vi "Create or Load Experiment Dialog.vi"(8 "error in (no error)":errorcluster) -> (0 "error out":errorcluster, 1 "Cancelled?":bool, 2 "Experimental File Cluster":T1, 3 "Experiment File Path":path, 4 "Experiment File Extension":string, 5 "Experiment Name":string)   [LabVIEW 2020, in "Experiment Manager.lvlib"]
uses:
  Experiment Manager.lvlib
  Experiment File/Experiment File Cluster.ctl
  Plugin Servers/Controller/Minimal Controller Cluster.ctl
  Plugin Servers/Parameter to Hardware Map/Minimal Map.ctl
  Plugin Servers/Parameter to Hardware Map/Minimal Pair Cluster.ctl
  UI Data.ctl
  User Preferences/User Preferences File.lvclass
  Sub VIs/Message Queue/Enqueue Message (Single).vi
  <vilib>/Utility/error.llb/Error Cluster From Error Code.vi
  <vilib>/ErrorRing/Error Ring.xnode
  Sub VIs/Message Queue/test Message Queue.lvlib
  User Event - Stop/User Event - Stop.lvlib
  Plugin Servers/Controller/Generic Plugin.lvclass
  Experiment File/Experiment File.lvlib
  Plugin Servers/Parameter to Hardware Map/Parameter to Hardware Map.lvclass
panel:
  in  "Continue Without Experiment Btn":bool
  in  "Load Experiment Btn":bool
  in  "New Experiment Btn":bool
  in  "Clear Recent Experiments Button":bool
  in  "Recent Experiments Listbox":i32(listbox)
  # "Create or Load Experiment"
  # "Experiment Options"
  # "Recent Experiments"
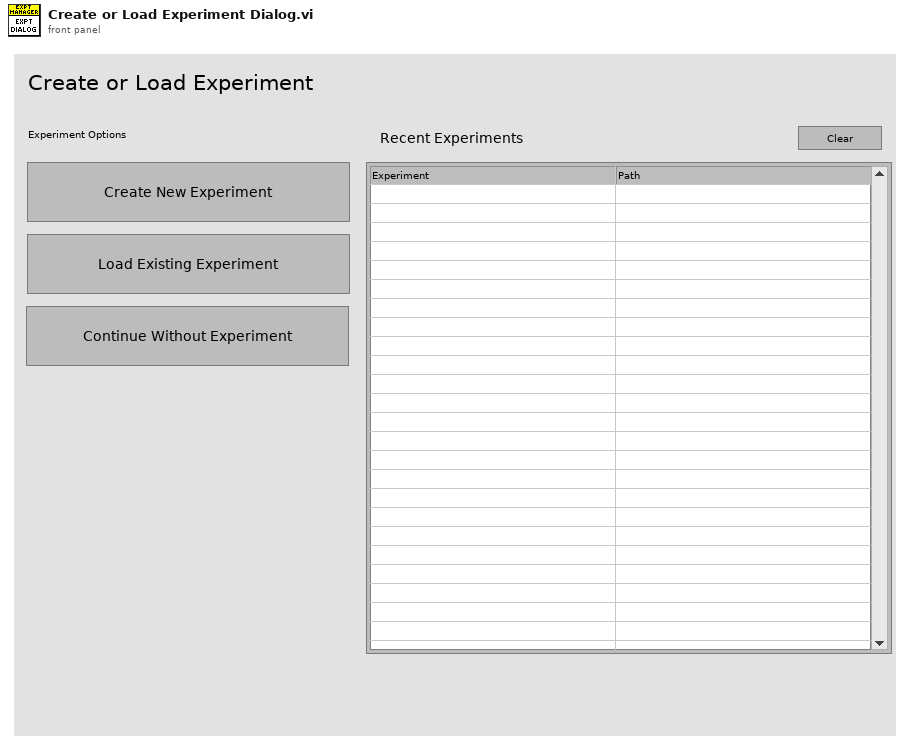
[diagram p1: front panel]
types:
  T1 = typedef "Experiment File.lvlib/Experiment File Cluster.ctl" = cluster{"Hardware List":T2[], "Optimizer List":T2[], "Analyzer List":T2[], "Parameter to Hardware Map":T3}
  T2 = typedef "Generic Plugin.lvclass/Minimal Controller Cluster.ctl" = cluster{"Name":string, "Controller Type":string, "Control Panel Path":string, "Resource":string}
  T3 = typedef "Parameter to Hardware Map.lvclass/Minimal Map.ctl" = T4[]
  T4 = typedef "Parameter to Hardware Map.lvclass/Minimal Pair Cluster.ctl" = cluster{"key":string, "values":T2[]}
  T5 = typedef "Experiment Manager.lvlib/UI Data.ctl" = cluster{"New Project Btn":refnum<vi>, "Load Project Btn":refnum<vi>, "Cancelled?":bool, "Experiment File Path":path, "Experiment File":T1, "Experiment Directory":path, "Experiment Name":string, "Experiment File Extension":string, "User Preferences File":refnum<class "User Preferences File.lvclass">, "Recent Experiments Listbox":refnum<vi>}
  T6 = enum32{"Invalid", "Standard", "Closed", "Hidden", "Minimized", "Maximized"}
  T7 = typedef "User Preferences File.lvclass/User Preferences Cluster.ctl" = cluster{"Max Recent Experiments":dbl, "Recent Experiments":string[]}
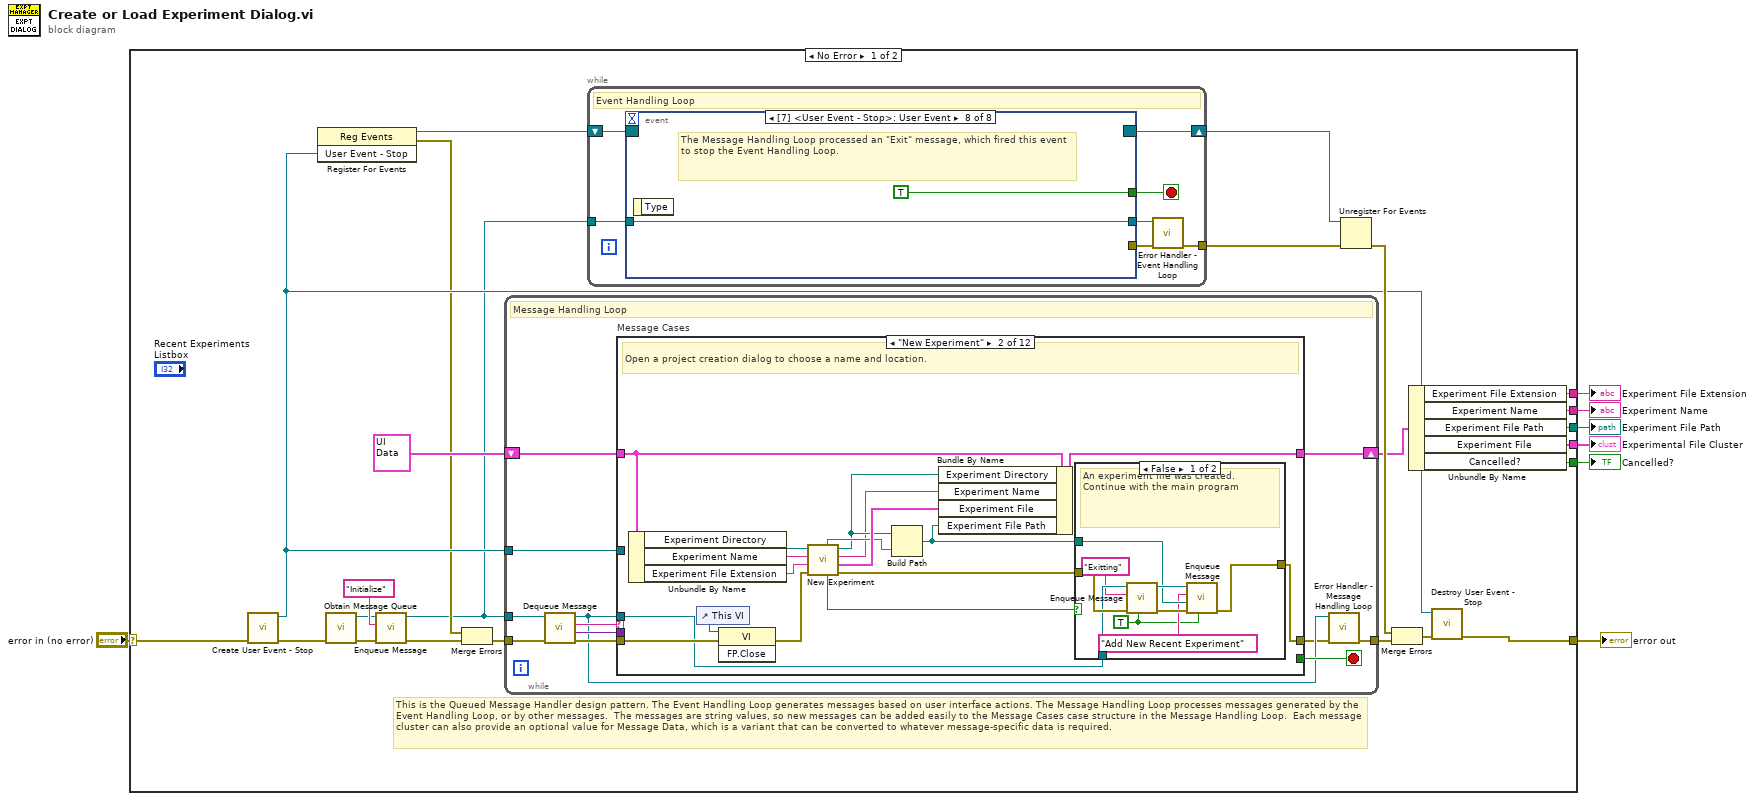
[diagram p0: block diagram]
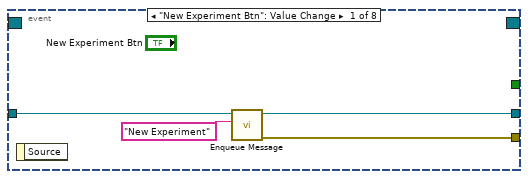
[diagram p2: hidden frame]
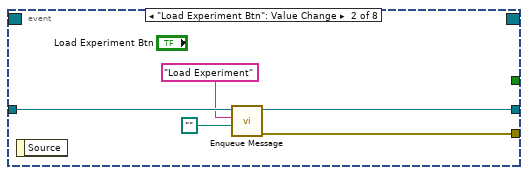
[diagram p3: hidden frame]
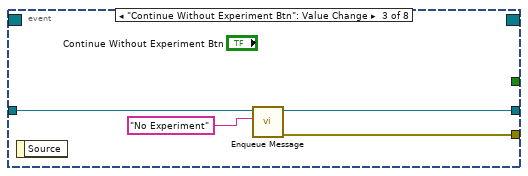
[diagram p4: hidden frame]
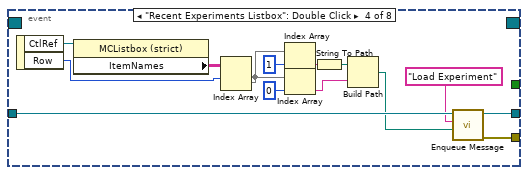
[diagram p5: hidden frame]
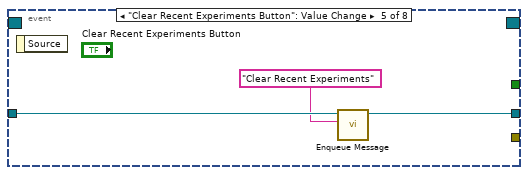
[diagram p6: hidden frame]
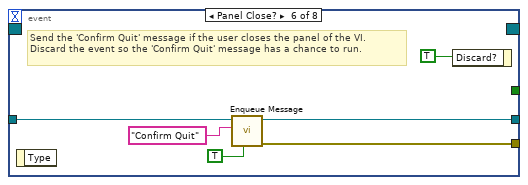
[diagram p7: hidden frame]
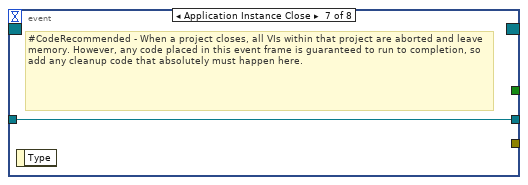
[diagram p8: hidden frame]
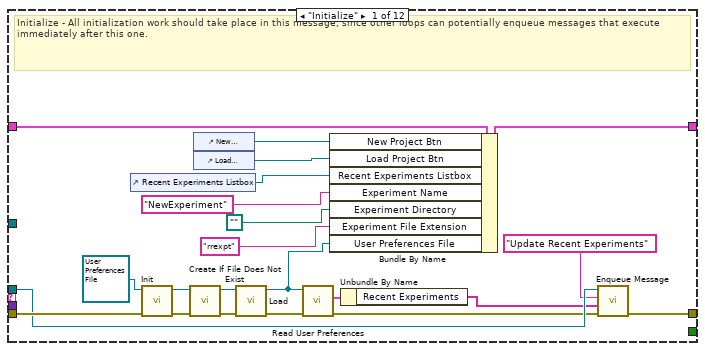
[diagram p9: hidden frame]
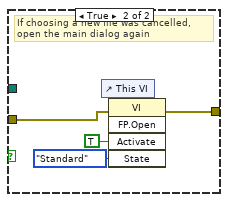
[diagram p10: hidden frame]
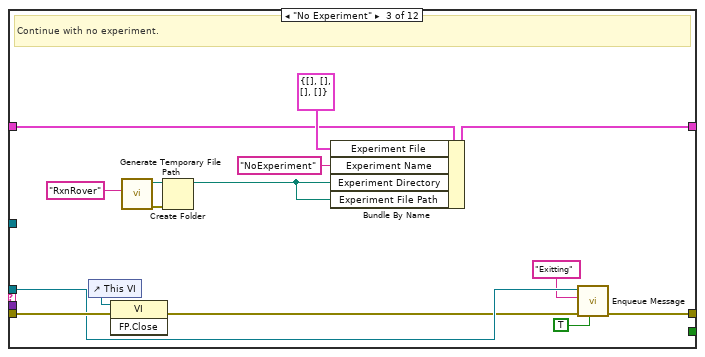
[diagram p11: hidden frame]
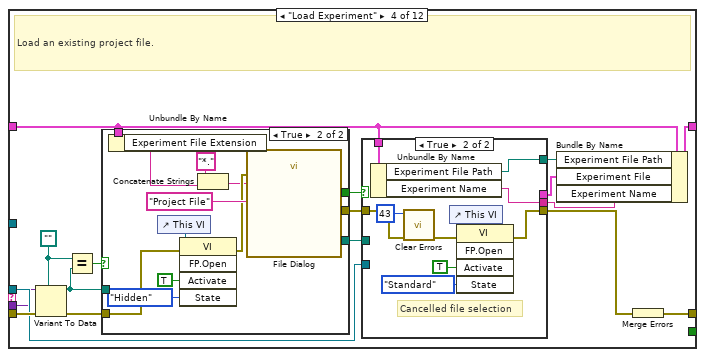
[diagram p12: hidden frame]
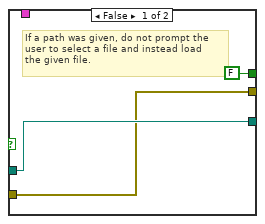
[diagram p13: hidden frame]
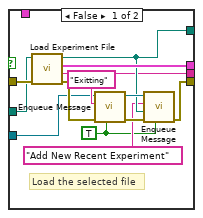
[diagram p14: hidden frame]
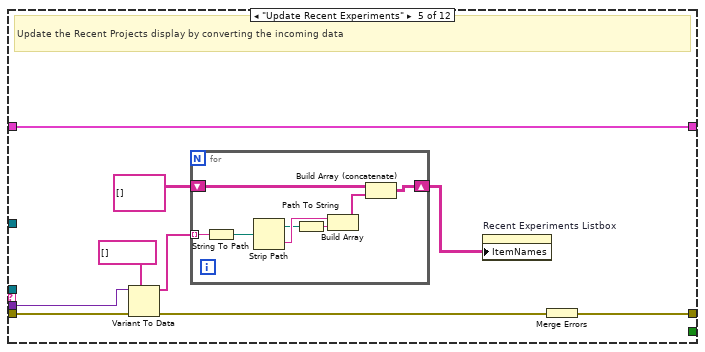
[diagram p15: hidden frame]
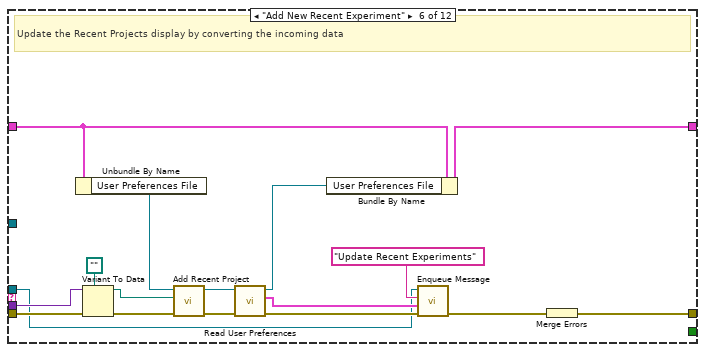
[diagram p16: hidden frame]
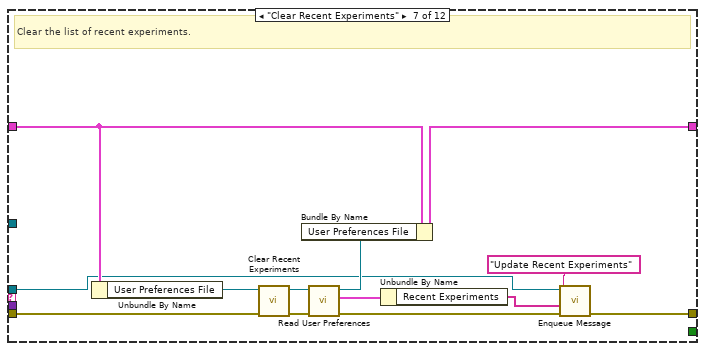
[diagram p17: hidden frame]
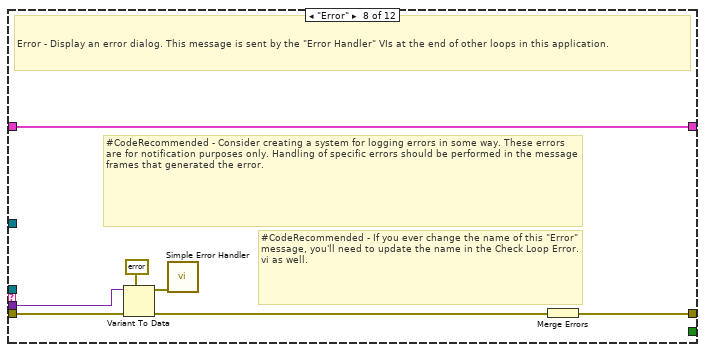
[diagram p18: hidden frame]
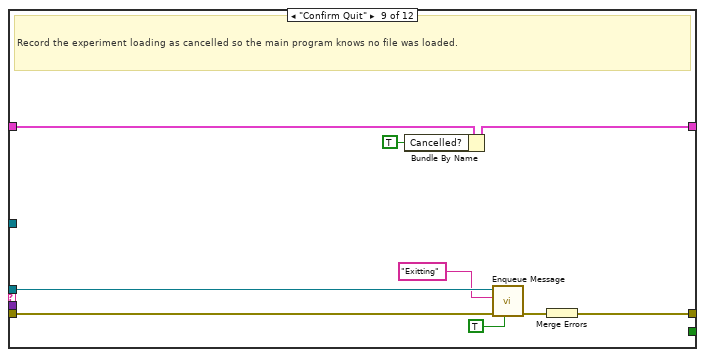
[diagram p19: hidden frame]
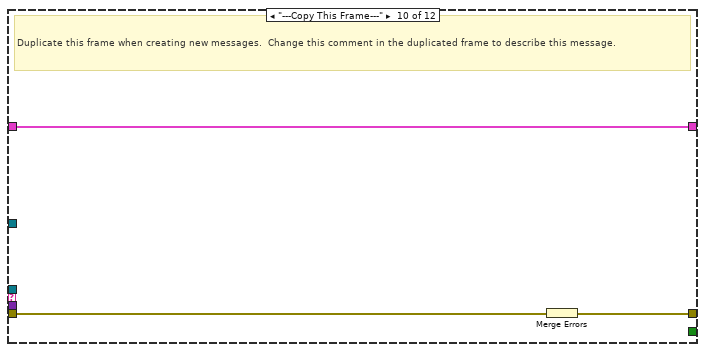
[diagram p20: hidden frame]
diagram:
  n1 = case shown="No Error" "error in (no error)" {
    selector: "error in (no error)" -> [w11 w307]
    tunnel: [w15 w307] -> w1
    tunnel: [w13 T1 {"Hardware List"=[], "Optimizer List"=[], "Analyzer List"=[], "Parameter to Hardware Map"=[]} ("File")] -> w7
    tunnel: [w12 TRUE ("Cancelled?")] -> w6
    tunnel: [w10 path ""] -> w4
    tunnel: [w9 w303] -> w3
    tunnel: [w8 w303] -> w2
    frame No Error {
      # "This is the Queued Message Handler design pattern. The Event Handling Loop generates messages based on user interface actions. The Message Handling Loop processes messages generated by the Event Handling Loop, or by other messages.  The messages are string values, so new messages can be added easily to the Message Cases case structure in the Message Handling Loop.  Each message cluster can also provide an optional value for Message Data, which is a variant that can be converted to whatever message-specific data is required."
      n2 = call "Create User Event - Stop.vi"("error in (no error)"=w11) -> ("error out"=w21:errorcluster, "User Event - Stop"=w24:refnum<user-event>)  [unwired: 9 in]
      n3 = register-events(w24) -> (reference out=w25:refnum<event-registration>, error out=w22:errorcluster)  [unwired: 2 in]
      n4 = call "Obtain Message Queue.vi"("error in (no error)"=w21) -> ("error out"=w20:errorcluster, "Message Queue"=w17:refnum<queue>)  [unwired: 9 in]
      n5 = call-poly "Enqueue Message.vi"("error in (no error)"=w20, "Message"="Initialize", "Message Queue"=w17) -> ("error out"=w19:errorcluster, "dup Message Queue"=w16:refnum<queue>)  [unwired: 7 in]
      n6 = Merge Errors(w22, w19) -> (w23:errorcluster)
      n7 = while {
        tunnel: w16 -> [w81]
        shift-right: [w88] -> w14
        shift-left: T5 {"New Project Btn"=refnum, "Load Project Btn"=refnum, "Cancelled?"=FALSE, "Experiment File Path"=path "", "Experiment File"={"Hardware List"=[], "Optimizer List"=[], "Analyzer List"=[], "Parameter to Hardware Map"=[]}, "Experiment Directory"=path "", "Experiment Name"="", "Experiment File Extension"="", "User Preferences File"=refnum, "Recent Experiments Listbox"=refnum} ("Data Cluster") -> [w89]
        tunnel: w24 -> [w86]
        tunnel: w23 -> [w85]
        tunnel: [w79] -> w31
        stop <- w87 stop-if-true
        # "Message Handling Loop"
        n8 = call "Dequeue Message.vi"("error in (no error)"=w85, "Message Queue"=w81) -> ("error out"=w84:errorcluster, "Message Data"=w82:variant, "Message"=w83:string, "dup Message Queue"=w80:refnum<queue>)  [unwired: 6 in]
        n9 = case "Message Cases" shown="\"New Experiment\"" w83 {
          selector: w83 -> [_ _ _ _ _ _ _ _ _ _ _ w293]
          tunnel: w80 -> [w105 w122 w154 w164 _ w232 w250 _ w272 _ w292 _]
          tunnel: w84 -> [w110 w126 w155 w168 w220 w246 w260 w267 w276 w279 w286 _]
          tunnel: [w111 w123 w151 w174 w221 w247 w251 w261 w274 w277 w289 w294] -> w78
          tunnel: w89 -> [w109 w121 w145 w165 w222 w243 w259 w266 w275 w278 w282 w295]
          tunnel: [w108 w128 w157 w169 w222 w238 w257 w266 w269 w278 w282 w295] -> w88
          tunnel: [_ _ _ _ _ _ _ _ _ _ TRUE _] -> w87
          tunnel: w82 -> [_ _ _ w162 w219 w245 _ w265 _ _ w283 _]
          tunnel: w86 -> [_ _ _ _ _ _ _ _ _ _ w288 _]
          frame "Initialize" {
            # "Initialize - All initialization work should take place in this message, since other loops can potentially enqueue messages that execute immediately after this one."
            n10 = control-ref of="Recent Experiments Listbox"() -> (w93:refnum<vi>)
            n11 = call "Init.vi"("error in (no error)"=w110, "UserPreferencesFileManager in"=refnum<class "User Preferences File.lvclass"> refnum ("User Preferences File.lvclass")) -> ("error out"=w100:errorcluster, "UserPreferencesFileManager out"=w91:refnum<class "User Preferences File.lvclass">)  [unwired: 8 in]
            n12 = call "Create If File Does Not Exist.vi"("error in (no error)"=w100, "User Preferences File in"=w91) -> ("error out"=w92:errorcluster, "User Preferences File out"=w90:refnum<class "User Preferences File.lvclass">)  [unwired: 8 in]
            n13 = control-ref of="New Experiment Btn"() -> (w107:refnum<vi>)
            n14 = control-ref of="Load Experiment Btn"() -> (w106:refnum<vi>)
            n15 = call "Load.vi"("error in (no error)"=w92, "User Preferences File in"=w90) -> ("error out"=w98:errorcluster, "User Preferences File out"=w96:refnum<class "User Preferences File.lvclass">)  [unwired: 8 in]
            n16 = call-dynamic "Read User Preferences.vi"("error in (no error)"=w98, "User Preferences File in"=w96) -> ("error out"=w97:errorcluster, "User Preferences"=w95:T7)  [unwired: 7 in, 1 out]
            n17 = Bundle By Name(cluster=w109, "New Project Btn"=w107, "Load Project Btn"=w106, "Recent Experiments Listbox"=w93, "Experiment Name"="NewExperiment", "Experiment Directory"=path "", "Experiment File Extension"="rrexpt", "User Preferences File"=w96) -> (w108:T5)
            n18 = Unbundle By Name(w95) -> ("Recent Experiments"=w94:string[])
            n19 = call-poly "Enqueue Message.vi"("error in (no error)"=w97, "Message Data"=w94, "Message"="Update Recent Experiments", "Message Queue"=w105) -> ("error out"=w111:errorcluster)  [unwired: 6 in, 1 out]
          }
          frame "New Experiment" {
            # "Open a project creation dialog to choose a name and location."
            n20 = Unbundle By Name(w121) -> ("Experiment Directory"=w119:path, "Experiment Name"=w113:string, "Experiment File Extension"=w115:string)
            n21 = control-ref of="This VI"() -> (w127:refnum<vi>)
            n22 = invoke class="VI" method="FP.Close"(reference=w127, error in=w126) -> (error out=w125:errorcluster)  [unwired: 1 in, 2 out]
            n23 = call "New Experiment.vi"("error in (no error)"=w125, "Experiment File Extension"=w115, "Experiment Name in"=w113, "Experiment Location in"=w119) -> ("error out"=w124:errorcluster, "Experiment File Cluster"=w118:T1, "Experiment Name out"=w112:string, "Experiment Location out"=w116:path, "cancelled"=w120:bool, "Experiment filename out"=w117:string)  [unwired: 2 in]
            n24 = Build Path(base path=w116, name or relative path=w117) -> (appended path=w114:path)
            n25 = Bundle By Name(cluster=w121, "Experiment Directory"=w116, "Experiment Name"=w112, "Experiment File"=w118, "Experiment File Path"=w114) -> (w128:T5)
            n26 = case shown="False" w120 {
              tunnel: w124 -> [w137 w141]
              tunnel: [w133 w140] -> w123
              tunnel: w122 -> [w136 _]
              tunnel: w114 -> [w131 _]
              frame False {
                w129 = TRUE ("Priority Message? (F)")
                # "An experiment file was created. Continue with the main program"
                n27 = call-poly "Enqueue Message.vi"("Priority Message? (F)"=w129, "error in (no error)"=w137, "Message"="Exitting", "Message Queue"=w136) -> ("error out"=w134:errorcluster, "dup Message Queue"=w132:refnum<queue>)  [unwired: 6 in]
                n28 = call-poly "Enqueue Message.vi"("Priority Message? (F)"=w129, "error in (no error)"=w134, "Message Data"=w131, "Message"="Add New Recent Experiment", "Message Queue"=w132) -> ("error out"=w133:errorcluster)  [unwired: 5 in, 1 out]
              }
              frame True {
                # "If choosing a new file was cancelled, open the main dialog again"
                n29 = control-ref of="This VI"() -> (w142:refnum<vi>)
                n30 = invoke class="VI" method="FP.Open"(reference=w142, error in=w141, "Activate"=TRUE ("Activate?"), "State"=T6."Standard") -> (error out=w140:errorcluster)  [unwired: 1 in, 4 out]
              }
            }
          }
          frame "No Experiment" {
            # "Continue with no experiment."
            n31 = control-ref of="This VI"() -> (w156:refnum<vi>)
            n32 = invoke class="VI" method="FP.Close"(reference=w156, error in=w155) -> (error out=w147:errorcluster)  [unwired: 1 in, 2 out]
            n33 = call <vilib>:"Generate Temporary File Path.vi"("Temporary File Extension (tmp)"="RxnRover") -> ("error out"=w149:errorcluster, "Unique Temporary File Path"=w150:path)  [unwired: 9 in]
            n34 = Create Folder(path (use dialog)=w150, error in=w149) -> (created path=w143:path)  [unwired: 1 in, 2 out]
            n35 = Bundle By Name(cluster=w145, "Experiment File"=T1 {"Hardware List"=[], "Optimizer List"=[], "Analyzer List"=[], "Parameter to Hardware Map"=[]} ("Experiment File Cluster"), "Experiment Name"="NoExperiment", "Experiment Directory"=w143, "Experiment File Path"=w143) -> (w157:T5)
            n36 = call-poly "Enqueue Message.vi"("Priority Message? (F)"=TRUE, "error in (no error)"=w147, "Message"="Exitting", "Message Queue"=w154) -> ("error out"=w151:errorcluster)  [unwired: 6 in, 1 out]
          }
          frame "Load Experiment" {
            w160 = path ""
            # "Load an existing project file."
            n37 = Variant To Data(error in=w168, type=w160, Variant=w162) -> (data=w159:path, error out=w163:errorcluster)
            n38 = Equal?(x=w160, y=w159) -> (x = y?=w161:bool)
            n39 = case shown="True" w161 {
              tunnel: [FALSE ("cancelled") w189] -> w173
              tunnel: [w175 w188] -> w172
              tunnel: [w177 w187] -> w170
              tunnel: w163 -> [w175 w186]
              tunnel: w165 -> [_ w181]
              tunnel: w159 -> [w177 _]
              frame False {
                # "If a path was given, do not prompt the\nuser to select a file and instead load\nthe given file."
              }
              frame True {
                n40 = Unbundle By Name(w181) -> ("Experiment File Extension"=w179:string)
                n41 = control-ref of="This VI"() -> (w184:refnum<vi>)
                n42 = invoke class="VI" method="FP.Open"(reference=w184, error in=w186, "Activate"=TRUE ("Activate?"), "State"=T6."Hidden") -> (error out=w185:errorcluster)  [unwired: 1 in, 4 out]
                n43 = Concatenate Strings("*." ("pattern (all files)"), w179) -> (w180:string)
                n44 = call "File Dialog"("button label"="Project File", "error in"=w185, "pattern (all files)"=w180) -> ("selected path"=w187:path, "cancelled"=w189:bool, "error out"=w188:errorcluster)  [unwired: 9 in, 1 out]
              }
            }
            n45 = case shown="True" w173 {
              tunnel: w172 -> [w203 w208]
              tunnel: [w196 w210] -> w171
              tunnel: w170 -> [w202 _]
              tunnel: [w198 _] -> w167
              tunnel: w164 -> [w199 _]
              tunnel: [w194 w205] -> w166
              tunnel: w165 -> [_ w206]
              tunnel: [w191 w204] -> w158
              frame False {
                w192 = TRUE ("Priority Message? (F)")
                # "Load the selected file"
                n46 = call "Load Experiment File.vi"("error in (no error)"=w203, "Experiment File Path"=w202) -> ("error out"=w200:errorcluster, "Experiment Name"=w191:string, "Experiment File out"=w198:T1, "Experiment File Path out (duplicate)"=w194:path)  [unwired: 6 in]
                n47 = call-poly "Enqueue Message.vi"("Priority Message? (F)"=w192, "error in (no error)"=w200, "Message"="Exitting", "Message Queue"=w199) -> ("error out"=w197:errorcluster, "dup Message Queue"=w195:refnum<queue>)  [unwired: 6 in]
                n48 = call-poly "Enqueue Message.vi"("Priority Message? (F)"=w192, "error in (no error)"=w197, "Message Data"=w194, "Message"="Add New Recent Experiment", "Message Queue"=w195) -> ("error out"=w196:errorcluster)  [unwired: 5 in, 1 out]
              }
              frame True {
                # "Cancelled file selection"
                n49 = Unbundle By Name(w206) -> ("Experiment File Path"=w205:path, "Experiment Name"=w204:string)
                n50 = call <vilib>:"Clear Errors.vi"("error in (no error)"=w208, "specific error code to clear (0: all)"=43) -> ("error out"=w207:errorcluster)  [unwired: 4 in, 1 out]
                n51 = control-ref of="This VI"() -> (w213:refnum<vi>)
                n52 = invoke class="VI" method="FP.Open"(reference=w213, error in=w207, "Activate"=TRUE ("Activate?"), "State"=T6."Standard") -> (error out=w210:errorcluster)  [unwired: 1 in, 4 out]
              }
            }
            n53 = Bundle By Name(cluster=w165, "Experiment File Path"=w166, "Experiment File"=w167, "Experiment Name"=w158) -> (w169:T5)
            n54 = Merge Errors(w171) -> (w174:errorcluster)
          }
          frame "Update Recent Experiments" {
            # "Update the Recent Projects display by converting the incoming data"
            n55 = Variant To Data(error in=w220, type=string[] [], Variant=w219) -> (data=w216:string[], error out=w218:errorcluster)
            n56 = for {
              tunnel: w216 -> [w230] mode=indexing
              shift-right: [w228] -> w214
              shift-left: string[][] [] -> [w229]
              n57 = String To Path(string=w230) -> (path=w223:path)
              n58 = Strip Path(path=w223) -> (stripped path=w226:path, name=w227:string)
              n59 = Path To String(path=w226) -> (string=w224:string)
              n60 = Build Array(w227, w224) -> (w225:string[])
              n61 = Build Array (concatenate)(w229, w225) -> (w228:string[][])
            }
            n62 = property on="Recent Experiments Listbox" class="MCListbox (strict)"("ItemNames"=w214) -> ()  [unwired: 2 in, 2 out]
            n63 = Merge Errors(w218) -> (w221:errorcluster)
          }
          frame "Add New Recent Experiment" {
            # "Update the Recent Projects display by converting the incoming data"
            n64 = Unbundle By Name(w243) -> ("User Preferences File"=w241:refnum<class "User Preferences File.lvclass">)
            n65 = Variant To Data(error in=w246, type=path "", Variant=w245) -> (data=w231:path, error out=w242:errorcluster)
            n66 = call "Add Recent Project.vi"("error in (no error)"=w242, "New Recent Experiment path"=w231, "User Preferences File in"=w241) -> ("error out"=w240:errorcluster, "User Preferences File out"=w239:refnum<class "User Preferences File.lvclass">)  [unwired: 7 in]
            n67 = call-dynamic "Read User Preferences.vi"("error in (no error)"=w240, "User Preferences File in"=w239) -> ("error out"=w236:errorcluster, "User Preferences"=w234:T7, "User Preferences File out"=w237:refnum<class "User Preferences File.lvclass">)  [unwired: 7 in]
            n68 = Bundle By Name(cluster=w243, "User Preferences File"=w237) -> (w238:T5)
            n69 = call-poly "Enqueue Message.vi"("error in (no error)"=w236, "Message Data"=w234, "Message"="Update Recent Experiments", "Message Queue"=w232) -> ("error out"=w235:errorcluster)  [unwired: 6 in, 1 out]
            n70 = Merge Errors(w235) -> (w247:errorcluster)
          }
          frame "Clear Recent Experiments" {
            # "Clear the list of recent experiments."
            n71 = Unbundle By Name(w259) -> ("User Preferences File"=w258:refnum<class "User Preferences File.lvclass">)
            n72 = call "Clear Recent Experiments.vi"("error in (no error)"=w260, "User Preferences File in"=w258) -> ("error out"=w254:errorcluster, "User Preferences File out"=w256:refnum<class "User Preferences File.lvclass">)  [unwired: 8 in]
            n73 = call-dynamic "Read User Preferences.vi"("error in (no error)"=w254, "User Preferences File in"=w256) -> ("error out"=w252:errorcluster, "User Preferences"=w253:T7, "User Preferences File out"=w255:refnum<class "User Preferences File.lvclass">)  [unwired: 7 in]
            n74 = Bundle By Name(cluster=w259, "User Preferences File"=w255) -> (w257:T5)
            n75 = Unbundle By Name(w253) -> ("Recent Experiments"=w249:string[])
            n76 = call-poly "Enqueue Message.vi"("error in (no error)"=w252, "Message Data"=w249, "Message"="Update Recent Experiments", "Message Queue"=w250) -> ("error out"=w251:errorcluster)  [unwired: 6 in, 1 out]
          }
          frame "Error" {
            # "#CodeRecommended - If you ever change the name of this \"Error\" message, you'll need to update the name in the Check Loop Error.vi as well."
            # "#CodeRecommended - Consider creating a system for logging errors in some way. These errors are for notification purposes only. Handling of specific errors should be performed in the message frames that generated the error."
            # "Error - Display an error dialog. This message is sent by the \"Error Handler\" VIs at the end of other loops in this application."
            n77 = Variant To Data(error in=w267, type=errorcluster {"status"=FALSE, "code"=0, "source"=""} ("error constant"), Variant=w265) -> (data=w263:errorcluster, error out=w262:errorcluster)
            n78 = call <vilib>:"Simple Error Handler.vi"("error in (no error)"=w263) -> ()  [unwired: 4 in, 5 out]
            n79 = Merge Errors(w262) -> (w261:errorcluster)
          }
          frame "Confirm Quit" {
            # "Record the experiment loading as cancelled so the main program knows no file was loaded."
            n80 = Bundle By Name(cluster=w275, "Cancelled?"=TRUE) -> (w269:T5)
            n81 = call-poly "Enqueue Message.vi"("Priority Message? (F)"=TRUE, "error in (no error)"=w276, "Message"="Exitting", "Message Queue"=w272) -> ("error out"=w273:errorcluster)  [unwired: 6 in, 1 out]
            n82 = Merge Errors(w273) -> (w274:errorcluster)
          }
          frame "---Copy This Frame---" {
            # "Duplicate this frame when creating new messages.  Change this comment in the duplicated frame to describe this message."
            n83 = Merge Errors(w279) -> (w277:errorcluster)
          }
          frame "Exitting" {
            # "Stop the VI"
            # "Release the message queue reference"
            # "Exit - Exit the application."
            n84 = Unbundle By Name(w282) -> ("User Preferences File"=w281:refnum<class "User Preferences File.lvclass">)
            n85 = Variant To Data(type=errorcluster {"status"=FALSE, "code"=0, "source"=""} ("error constant"), Variant=w283) -> (data=w284:errorcluster)  [unwired: 1 in, 1 out]
            n86 = call <vilib>:"Simple Error Handler.vi"("error in (no error)"=w284) -> ()  [unwired: 4 in, 5 out]
            n87 = call "Fire User Event - Stop.vi"("User Event - Stop"=w288) -> ("error out"=w287:errorcluster)  [unwired: 10 in]
            n88 = call "Save.vi"("User Preferences File in"=w281) -> ("error out"=w280:errorcluster)  [unwired: 9 in, 1 out]
            n89 = Release Queue(queue=w292, error in (no error)=w286) -> (error out=w290:errorcluster)  [unwired: 1 in, 2 out]
            n90 = Merge Errors(w280, w287, w290) -> (w289:errorcluster)
          }
          frame Default {
            # "'Default' case only runs if there is a message that isn't defined in any of the other cases.  Output a programming error."
            n91 = xnode "Error Ring"("parameter 0"=w293) -> ("error out"=w294:errorcluster)
          }
        }
        n92 = call "Error Handler - Message Handling Loop.vi"("error in (no error)"=w78, "Message Queue"=w80) -> ("dup error in"=w79:errorcluster)  [unwired: 8 in, 1 out]
      }
      n93 = while {
        tunnel: w16 -> [w38]
        shift-right: [w36] -> w28
        shift-left: w25 -> [w37]
        tunnel: [w32] -> w26
        stop <- w34 stop-if-true
        # "Event Handling Loop"
        n94 = event shown="[7] <User Event - Stop>: User Event" {
          selector: w37 -> [_ _ _ _ _ _ _ _]
          dyn-events: [_ _ _ _ _ _ _ _] -> w36
          timeout: _ -> [_ _ _ _ _ _ _ _]
          tunnel: [_ _ _ _ _ _ _ TRUE ("Discard?")] -> w34
          tunnel: w38 -> [w42 w47 w50 w65 w68 w73 w75 w77]
          tunnel: [w39 w44 w48 w63 _ w72 _ _] -> w35
          tunnel: [w41 w46 w49 w64 w67 w71 w75 w77] -> w33
          event "New Experiment Btn": Value Change {
            n95 = event-data() -> ()  [unwired: 1 in, 1 out]
            n96 = call-poly "Enqueue Message.vi"("Message"="New Experiment", "Message Queue"=w42) -> ("error out"=w39:errorcluster, "dup Message Queue"=w41:refnum<queue>)  [unwired: 8 in]
          }
          event "Load Experiment Btn": Value Change {
            n97 = event-data() -> ()  [unwired: 1 in, 1 out]
            n98 = call-poly "Enqueue Message.vi"("Message Data"=path "", "Message"="Load Experiment", "Message Queue"=w47) -> ("error out"=w44:errorcluster, "dup Message Queue"=w46:refnum<queue>)  [unwired: 7 in]
          }
          event "Continue Without Experiment Btn": Value Change {
            n99 = event-data() -> ()  [unwired: 1 in, 1 out]
            n100 = call-poly "Enqueue Message.vi"("Message"="No Experiment", "Message Queue"=w50) -> ("error out"=w48:errorcluster, "dup Message Queue"=w49:refnum<queue>)  [unwired: 8 in]
          }
          event "Recent Experiments Listbox": Double Click {
            n101 = event-data() -> ("CtlRef"=w61:refnum<vi>, "Row"=w59:i32)  [unwired: 1 in]
            n102 = property class="MCListbox (strict)"(reference=w61) -> ("ItemNames"=w60:string[][])  [unwired: 1 in, 2 out]
            n103 = Index Array(array=w60, index (row)=w59) -> (element=w58:string[])  [unwired: 1 in]
            n104 = Index Array(array=w58, index=1) -> (element=w55:string)
            n105 = Index Array(array=w58, index=0) -> (element=w54:string)
            n106 = String To Path(string=w55) -> (path=w53:path)
            n107 = Build Path(base path=w53, name or relative path=w54) -> (appended path=w52:path)
            n108 = call-poly "Enqueue Message.vi"("Message Data"=w52, "Message"="Load Experiment", "Message Queue"=w65) -> ("error out"=w63:errorcluster, "dup Message Queue"=w64:refnum<queue>)  [unwired: 7 in]
          }
          event "Clear Recent Experiments Button": Value Change {
            n109 = event-data() -> ()  [unwired: 1 in, 1 out]
            n110 = call-poly "Enqueue Message.vi"("Message"="Clear Recent Experiments", "Message Queue"=w68) -> ("dup Message Queue"=w67:refnum<queue>)  [unwired: 8 in, 1 out]
          }
          event Panel Close? {
            # "Send the 'Confirm Quit' message if the user closes the panel of the VI. Discard the event so the 'Confirm Quit' message has a chance to run."
            n111 = event-data() -> ()  [unwired: 1 in, 1 out]
            n112 = call-poly "Enqueue Message.vi"("Priority Message? (F)"=TRUE, "Message"="Confirm Quit", "Message Queue"=w73) -> ("error out"=w72:errorcluster, "dup Message Queue"=w71:refnum<queue>)  [unwired: 7 in]
            n113 = event-data("Discard?"=TRUE) -> ()  [unwired: 1 in, 1 out]
          }
          event Application Instance Close {
            # "#CodeRecommended - When a project closes, all VIs within that project are aborted and leave memory. However, any code placed in this event frame is guaranteed to run to completion, so add any cleanup code that absolutely must happen here."
            n114 = event-data() -> ()  [unwired: 1 in, 1 out]
          }
          event User Event {
            # "The Message Handling Loop processed an \"Exit\" message, which fired this event to stop the Event Handling Loop."
            n115 = event-data() -> ()  [unwired: 1 in, 1 out]
          }
        }
        n116 = call "Error Handler - Event Handling Loop.vi"("error in (no error)"=w35, "Message Queue"=w33) -> ("dup error in"=w32:errorcluster)  [unwired: 8 in, 1 out]
      }
      n117 = Unregister For Events(event registration refnum=w28, error in=w26) -> (error out=w29:errorcluster)
      n118 = Merge Errors(w29, w31) -> (w30:errorcluster)
      n119 = Unbundle By Name(w14) -> ("Experiment File Extension"=w8:string, "Experiment Name"=w9:string, "Experiment File Path"=w10:path, "Experiment File"=w13:T1, "Cancelled?"=w12:bool)
      n120 = call "Destroy User Event - Stop.vi"("error in (no error)"=w30, "User Event - Stop"=w24) -> ("error out"=w15:errorcluster)  [unwired: 9 in]
    }
    frame Error {
      w303 = ""
    }
  }
  "error out" <- w1
  "Experimental File Cluster" <- w7
  "Cancelled?" <- w6
  "Experiment File Path" <- w4
  "Experiment Name" <- w3
  "Experiment File Extension" <- w2
